vi "EnableDisable Custom Device.vi"(8 "error in (no error)":errorcluster, 11 "Node Ptr":u64 format="%.0x") -> (0 "error out":errorcluster)   [LabVIEW 2013, in "MUX Custom Device.lvlib"]
uses:
  MUX Custom Device.lvlib
  MUX Global.vi
  <vilib>/NI Veristand/Custom Device API/Custom Device API.lvlib
  <vilib>/NI Veristand/Custom Device Tools/Custom Device Utility Library/Custom Device Utility Library.lvlib
panel:
  in  "Tag":string
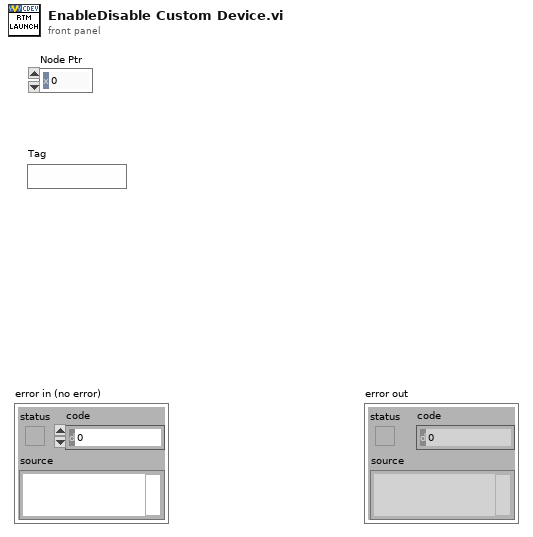
[diagram p1: front panel]
types:
  T1 = typedef "Custom Device API.lvlib/Custom Device Item Ref.ctl" = u64
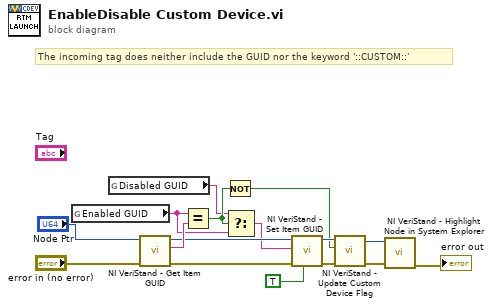
[diagram p0: block diagram]
diagram:
  # "The incoming tag does neither include the GUID nor the keyword '::CUSTOM::'"
  n1 = global read "MUX Global.vi" "Enabled GUID"() -> (w5:string)
  n2 = global read "MUX Global.vi" "Disabled GUID"() -> (w6:string)
  n3 = call <vilib>:"NI VeriStand - Get Item GUID.vi"("error in (no error)"="error in (no error)", "Item Ref in"="Node Ptr") -> ("error out"=w14:errorcluster, "GUID"=w16:string, "Item Ref out"=w13:T1)  [unwired: 7 in]
  n4 = Equal?(x=w5, y=w16) -> (x = y?=w9:bool)
  n5 = Not(x=w9) -> (.not. x?=w8:bool)
  n6 = Select(t=w6, s=w9, f=w5) -> (s? t:f=w12:string)
  n7 = call <vilib>:"NI VeriStand - Set Item GUID.vi"("Refresh System Explorer Tree? (F)"=TRUE, "error in (no error)"=w14, "GUID"=w12, "Item Ref in"=w13) -> ("error out"=w11:errorcluster, "Item Ref out"=w10:T1)  [unwired: 6 in]
  n8 = call <vilib>:"NI VeriStand - Update Custom Device Flag.vi"("error in (no error)"=w11, "Is Custom Device Active?"=w8, "Device Ref in"=w10) -> ("error out"=w3:errorcluster, "Device Ref out"=w2:T1)  [unwired: 7 in]
  n9 = call <vilib>:"NI VeriStand - Highlight Node in System Explorer.vi"("error in (no error)"=w3, "Item Ref in"=w2) -> ("error out"=→"error out":errorcluster)  [unwired: 8 in, 1 out]
